vi "Log Read.vi"() -> ()   [LabVIEW 2026, in "PXI_Common.lvlib"]
uses:
  PXI_Common.lvlib
panel:
  out "Log Table":string[][](table)
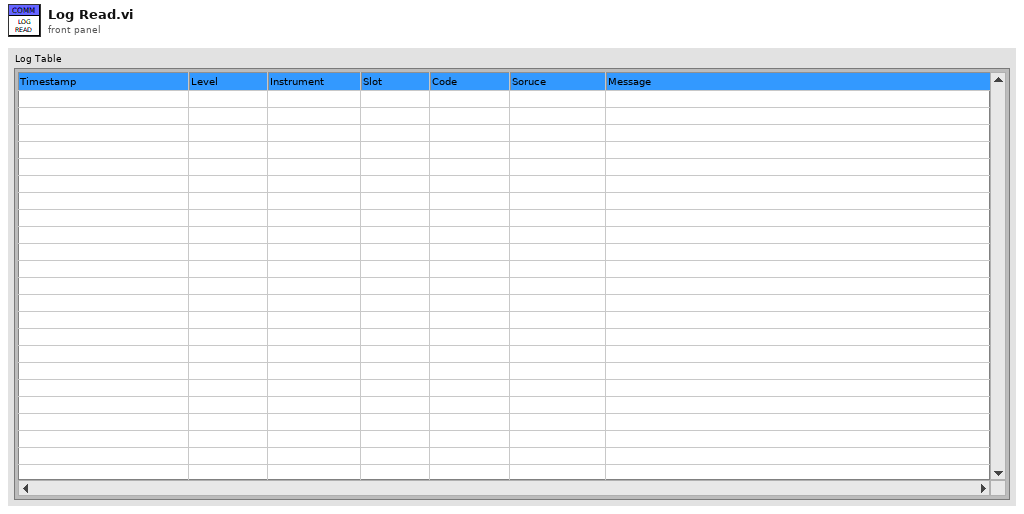
[diagram p1: front panel]
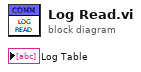
[diagram p0: block diagram]
diagram:
